vi "DUAL GAUGE-Driver Core.vi"(0 "Referenz in":refnum<visa-resource-name>, 1 "Write/Read":bool, 5 "Command":string, 11 "Fehler (Eingang)":errorcluster, 12 "Timeout [ms]":u32=600 min=1 max=40000 step=1, 13 "Retry (3)":i32=3 min=1 max=20000 step=1) -> (4 "Referenz out":refnum<visa-resource-name>, 8 "String Out":string, 15 "Cluster (Ausgang)":errorcluster)   [LabVIEW 2013, in "Dual Gauge.lvlib"]
uses:
  Dual Gauge.lvlib
panel:
  in  "ENQ [\\05]":string="\u0005"
  in  "NAK [\\15]":string="\u0015"
  in  "ACK [\\06]":string="\u0006"
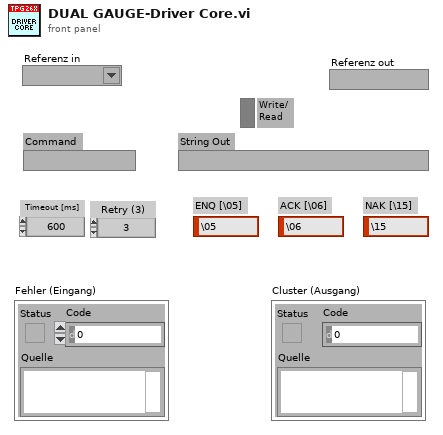
[diagram p1: front panel]
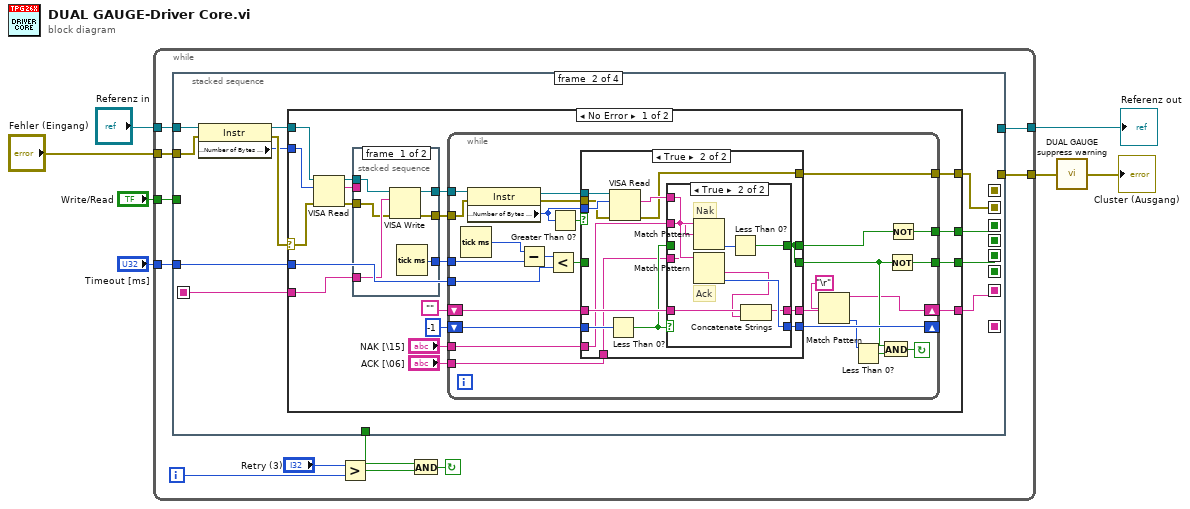
[diagram p0: block diagram]
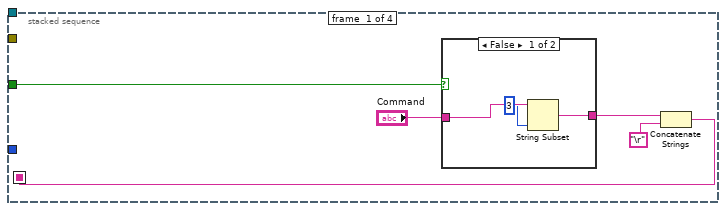
[diagram p2: hidden frame]
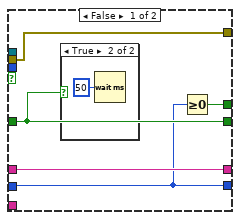
[diagram p4: hidden frame]
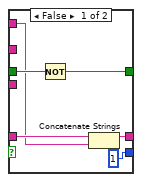
[diagram p6: hidden frame]
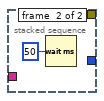
[diagram p7: hidden frame]
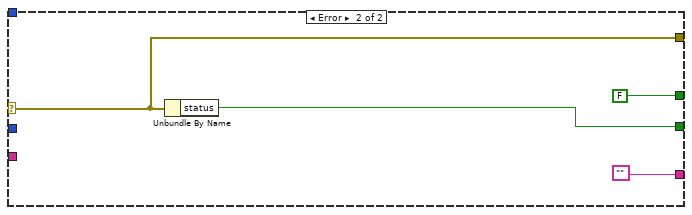
[diagram p8: hidden frame]
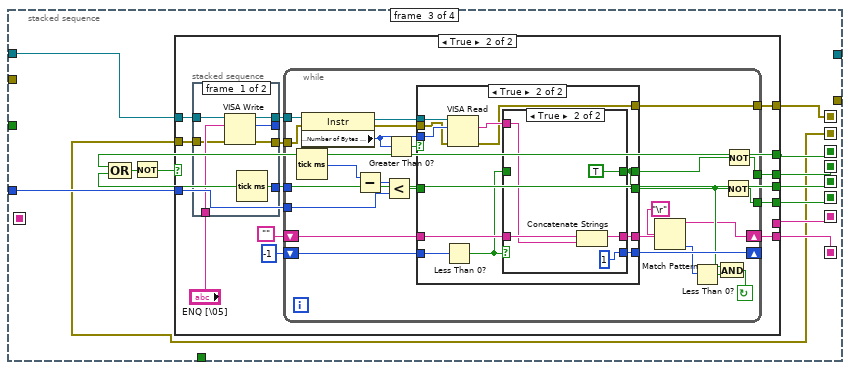
[diagram p9: hidden frame]
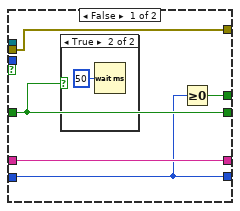
[diagram p11: hidden frame]
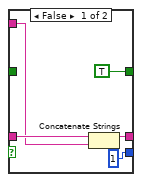
[diagram p13: hidden frame]
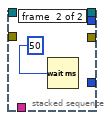
[diagram p14: hidden frame]
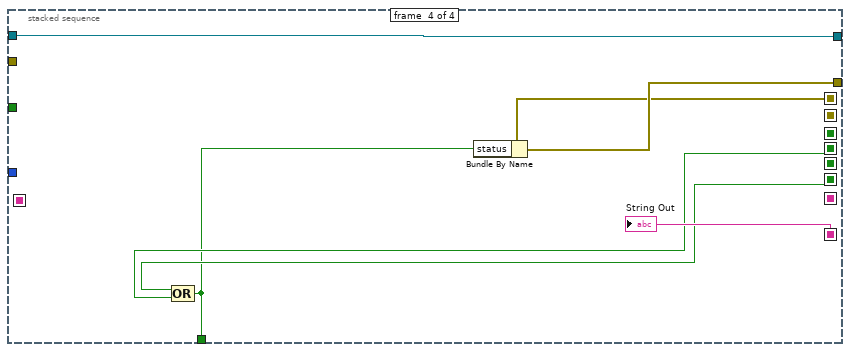
[diagram p15: hidden frame]
diagram:
  n1 = while {
    tunnel: "Write/Read" -> [w12]
    tunnel: "Timeout [ms]" -> [w18]
    tunnel: "Referenz in" -> [w11]
    tunnel: "Fehler (Eingang)" -> [w10]
    tunnel: [w9] -> w3
    tunnel: [w8] -> w2
    i -> [w16]
    stop <- w13 continue-if-true
    n2 = stacked-sequence {
      seq-local: [w23 _ _ _] -> [_ w36 _ _]
      seq-local: [_ w38 _ _] -> [_ _ w133 _]
      seq-local: [_ w34 _ _] -> [_ _ w135 _]
      seq-local: [_ w35 _ _] -> [_ _ w134 _]
      seq-local: [_ _ w140 _] -> [_ _ _ w224]
      seq-local: [_ _ w139 _] -> [_ _ _ w222]
      seq-local: [_ _ w138 _] -> [_ _ _ w225]
      seq-local: [_ w28 _ _] -> [_ _ w131 _]
      seq-local: [_ _ w130 _] -> [_ _ _ w219]
      tunnel: w18 -> [_ w37 w141 _]
      tunnel: [_ _ _ w221] -> w14
      tunnel: w12 -> [w22 _ _ _]
      tunnel: w11 -> [_ w33 w132 w223]
      tunnel: w10 -> [_ w31 _ _]
      tunnel: [_ _ _ w223] -> w9
      tunnel: [_ _ _ w220] -> w8
      frame #0 {
        n3 = case shown="False" w22 {
          tunnel: "Command" -> [w26 w27]
          tunnel: [w25 w27] -> w21
          frame False {
            n4 = String Subset(string=w26, length (rest)=u8 3 ("t")) -> (substring=w25:string)  [unwired: 1 in]
          }
          frame True {
          }
        }
        n5 = Concatenate Strings(w21, "\r") -> (w23:string)
      }
      frame #1 {
        n6 = property class="Instr"(reference=w33, error in=w31) -> (reference out=w29:refnum<visa-resource-name>, error out=w32:errorcluster, "Serial Settings:Number of Bytes at Serial Port"=w30:u32)
        n7 = case shown="No Error" w32 {
          selector: w32 -> [w45 w127]
          tunnel: [w57 FALSE] -> w34
          tunnel: [w56 w126] -> w35
          tunnel: w36 -> [w52 _]
          tunnel: w37 -> [w51 _]
          tunnel: [w49 ""] -> w38
          tunnel: w30 -> [w46 _]
          tunnel: w29 -> [w47 _]
          tunnel: [w39 w127] -> w28
          frame No Error {
            n8 = VISA Read(VISA resource name=w47, byte count=w46, error in (no error)=w45) -> (VISA resource name out=w44:refnum<visa-resource-name>, read buffer=w43:string, error out=w42:errorcluster)  [unwired: 1 out]
            n9 = stacked-sequence {
              tunnel: w52 -> [w123 _]
              tunnel: [w124 _] -> w50
              tunnel: w44 -> [w121 _]
              tunnel: w43 -> [_ _]
              tunnel: w42 -> [w122 _]
              tunnel: [w120 _] -> w41
              tunnel: [w119 _] -> w40
              frame #0 {
                n10 = VISA Write(VISA resource name=w121, write buffer=w123, error in (no error)=w122) -> (VISA resource name out=w119:refnum<visa-resource-name>, error out=w120:errorcluster)  [unwired: 1 out]
                n11 = Tick Count (ms)() -> (millisecond timer value=w124:u32)
              }
              frame #1 {
                n12 = Wait (ms)(milliseconds to wait=u32 50) -> ()  [unwired: 1 out]
              }
            }
            n13 = while {
              tunnel: "ACK [\\06]" -> [w69]
              tunnel: "NAK [\\15]" -> [w70]
              tunnel: [w71] -> w57
              tunnel: [w73] -> w56
              shift-left: -1 -> [w77]
              shift-right: [w76] -> _
              shift-left: "" -> [w78]
              shift-right: [w67] -> w49
              tunnel: w50 -> [w79]
              tunnel: w51 -> [w83]
              tunnel: w41 -> [w61]
              tunnel: w40 -> [w62]
              tunnel: [w58] -> w39
              stop <- w75 continue-if-true
              n14 = Tick Count (ms)() -> (millisecond timer value=w80:u32)
              n15 = property class="Instr"(reference=w62, error in=w61) -> (reference out=w60:refnum<visa-resource-name>, error out=w59:errorcluster, "Serial Settings:Number of Bytes at Serial Port"=w63:u32)
              n16 = Subtract(x=w80, y=w79) -> (x-y=w84:u32)
              n17 = Less?(x=w84, y=w83) -> (x < y?=w81:bool)
              n18 = Greater Than 0?(x=w63) -> (x > 0?=w82:bool)
              n19 = case shown="True" w82 {
                tunnel: w63 -> [_ w94]
                tunnel: w81 -> [w88 _]
                tunnel: w78 -> [w89 w101]
                tunnel: w77 -> [w86 w102]
                tunnel: [w86 w100] -> w76
                tunnel: [w89 w99] -> w68
                tunnel: [w88 w95] -> w74
                tunnel: [w87 w95] -> w72
                tunnel: w70 -> [_ w97]
                tunnel: w69 -> [_ w96]
                tunnel: w60 -> [_ w93]
                tunnel: w59 -> [w85 w92]
                tunnel: [w85 w91] -> w58
                frame False {
                  n20 = case shown="True" w88 {
                    frame False {
                    }
                    frame True {
                      n21 = Wait (ms)(milliseconds to wait=u32 50) -> ()  [unwired: 1 out]
                    }
                  }
                  n22 = Greater Or Equal To 0?(x=w86) -> (x >= 0?=w87:bool)
                }
                frame True {
                  n23 = Less Than 0?(x=w102) -> (x < 0?=w98:bool)
                  n24 = VISA Read(VISA resource name=w93, byte count=w94, error in (no error)=w92) -> (read buffer=w103:string, error out=w91:errorcluster)  [unwired: 2 out]
                  n25 = case shown="True" w98 {
                    tunnel: w103 -> [w104 w115]
                    tunnel: w101 -> [w109 w118]
                    tunnel: [1 w117] -> w100
                    tunnel: [w108 w116] -> w99
                    tunnel: [w105 w113] -> w95
                    tunnel: w98 -> [w106 _]
                    tunnel: w97 -> [_ w111]
                    tunnel: w96 -> [_ w110]
                    frame False {
                      n26 = Not(x=w106) -> (.not. x?=w105:bool)
                      n27 = Concatenate Strings(w109, w104) -> (w108:string)
                    }
                    frame True {
                      # "Ack"
                      # "Nak"
                      n28 = Match Pattern(string=w115, regular expression=w111) -> (offset past match=w114:i32)  [unwired: 1 in, 3 out]
                      n29 = Match Pattern(string=w115, regular expression=w110) -> (after substring=w112:string, offset past match=w117:i32)  [unwired: 1 in, 2 out]
                      n30 = Less Than 0?(x=w114) -> (x < 0?=w113:bool)
                      n31 = Concatenate Strings(w118, w112) -> (w116:string)
                    }
                  }
                }
              }
              n32 = Match Pattern(string=w68, regular expression="\r") -> (before substring=w67:string, offset past match=w64:i32)  [unwired: 1 in, 2 out]
              n33 = Less Than 0?(x=w64) -> (x < 0?=w65:bool)
              n34 = And(x=w74, y=w65) -> (x .and. y?=w75:bool)
              n35 = Not(x=w74) -> (.not. x?=w73:bool)
              n36 = Not(x=w72) -> (.not. x?=w71:bool)
            }
          }
          frame Error {
            n37 = Unbundle By Name(w127) -> ("status"=w126:bool)
          }
        }
      }
      frame #2 {
        n38 = Compound Arithmetic op=OR(w135, w134) -> (w137:bool)
        n39 = Not(x=w137) -> (.not. x?=w136:bool)
        n40 = case shown="True" w136 {
          tunnel: w141 -> [_ w157]
          tunnel: [w145 w153] -> w140
          tunnel: [w144 w152] -> w139
          tunnel: [w143 w151] -> w138
          tunnel: w135 -> [w145 _]
          tunnel: w134 -> [w144 _]
          tunnel: w133 -> [w143 _]
          tunnel: w132 -> [_ w150]
          tunnel: w131 -> [w142 w149]
          tunnel: [w142 w146] -> w130
          frame False {
          }
          frame True {
            n41 = stacked-sequence {
              tunnel: "ENQ [\\05]" -> [w216 _]
              tunnel: [w217 _] -> w156
              tunnel: w150 -> [w215 _]
              tunnel: [w214 _] -> w148
              tunnel: [w213 _] -> _
              tunnel: [w212 _] -> w147
              tunnel: w149 -> [w211 _]
              frame #0 {
                n42 = VISA Write(VISA resource name=w215, write buffer=w216, error in (no error)=w211) -> (VISA resource name out=w214:refnum<visa-resource-name>, return count=w213:u32, error out=w212:errorcluster)
                n43 = Tick Count (ms)() -> (millisecond timer value=w217:u32)
              }
              frame #1 {
                n44 = Wait (ms)(milliseconds to wait=u32 50) -> ()  [unwired: 1 out]
              }
            }
            n45 = while {
              tunnel: [w165] -> w152
              tunnel: [w166] -> w153
              shift-left: -1 -> [w176]
              shift-right: [w175] -> _
              shift-left: "" -> [w177]
              shift-right: [w170] -> w151
              tunnel: w156 -> [w178]
              tunnel: w157 -> [w182]
              tunnel: w148 -> [w164]
              tunnel: w147 -> [w163]
              tunnel: [w159] -> w146
              stop <- w174 continue-if-true
              n46 = Tick Count (ms)() -> (millisecond timer value=w179:u32)
              n47 = property class="Instr"(reference=w164, error in=w163) -> (reference out=w161:refnum<visa-resource-name>, error out=w160:errorcluster, "Serial Settings:Number of Bytes at Serial Port"=w162:u32)
              n48 = Subtract(x=w179, y=w178) -> (x-y=w183:u32)
              n49 = Less?(x=w183, y=w182) -> (x < y?=w180:bool)
              n50 = Greater Than 0?(x=w162) -> (x > 0?=w181:bool)
              n51 = case shown="True" w181 {
                tunnel: w162 -> [_ w193]
                tunnel: w180 -> [w187 _]
                tunnel: w177 -> [w188 w198]
                tunnel: w176 -> [w185 w199]
                tunnel: [w185 w197] -> w175
                tunnel: [w188 w196] -> w171
                tunnel: [w187 w194] -> w173
                tunnel: [w186 w194] -> w172
                tunnel: w161 -> [_ w192]
                tunnel: w160 -> [w184 w191]
                tunnel: [w184 w190] -> w159
                frame False {
                  n52 = case shown="True" w187 {
                    frame False {
                    }
                    frame True {
                      n53 = Wait (ms)(milliseconds to wait=u32 50) -> ()  [unwired: 1 out]
                    }
                  }
                  n54 = Greater Or Equal To 0?(x=w185) -> (x >= 0?=w186:bool)
                }
                frame True {
                  n55 = Less Than 0?(x=w199) -> (x < 0?=w195:bool)
                  n56 = VISA Read(VISA resource name=w192, byte count=w193, error in (no error)=w191) -> (read buffer=w200:string, error out=w190:errorcluster)  [unwired: 2 out]
                  n57 = case shown="True" w195 {
                    tunnel: w200 -> [w202 w208]
                    tunnel: w198 -> [w205 w210]
                    tunnel: [1 1] -> w197
                    tunnel: [w204 w209] -> w196
                    tunnel: [TRUE TRUE] -> w194
                    tunnel: w195 -> [_ _]
                    frame False {
                      n58 = Concatenate Strings(w205, w202) -> (w204:string)
                    }
                    frame True {
                      n59 = Concatenate Strings(w210, w208) -> (w209:string)
                    }
                  }
                }
              }
              n60 = Match Pattern(string=w171, regular expression="\r") -> (before substring=w170:string, offset past match=w167:i32)  [unwired: 1 in, 2 out]
              n61 = Less Than 0?(x=w167) -> (x < 0?=w168:bool)
              n62 = And(x=w173, y=w168) -> (x .and. y?=w174:bool)
              n63 = Not(x=w173) -> (.not. x?=w165:bool)
              n64 = Not(x=w172) -> (.not. x?=w166:bool)
            }
          }
        }
      }
      frame #3 {
        n65 = Compound Arithmetic op=OR(w222, w224) -> (w221:bool)
        n66 = Bundle By Name(cluster=w219, "status"=w221) -> (w220:errorcluster)
        "String Out" <- w225
      }
    }
    n67 = Greater?(x="Retry (3)", y=w16) -> (0:w15:bool)
    n68 = And(x=w14, y=w15) -> (x .and. y?=w13:bool)
  }
  "Referenz out" <- w3
  n69 = call "DUAL GAUGE suppress warning.vi"("error in"=w2) -> ("error out"=→"Cluster (Ausgang)":errorcluster)
